vi "ConvertTriggerEventsToEventList.vi"(11 "Trigger Events":enum16{"Source", "Delay", "Sense", "None"}[](array[ring])) -> (3 "Event List":string)   [LabVIEW 2012, in "Keithley-6482.lvlib"]
uses:
  Keithley-6482.lvlib
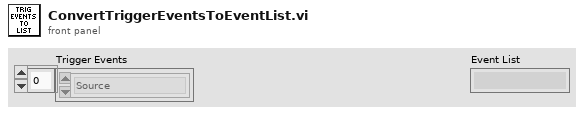
[diagram p1: front panel]
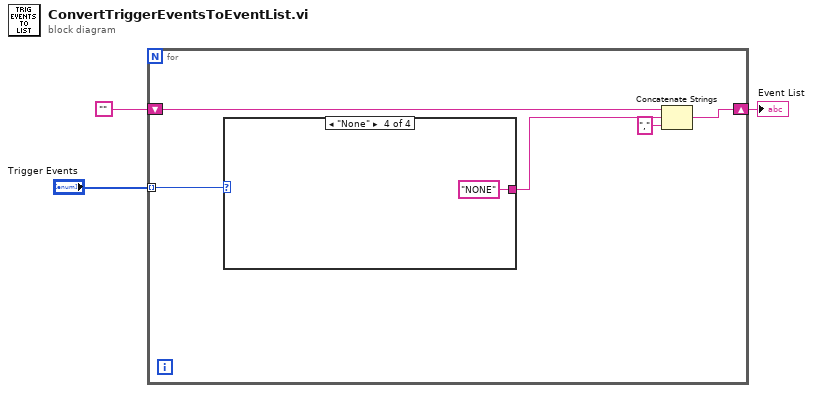
[diagram p0: block diagram]
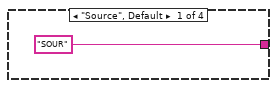
[diagram p2: hidden frame]
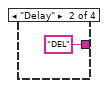
[diagram p3: hidden frame]
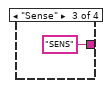
[diagram p4: hidden frame]
diagram:
  n1 = for {
    tunnel: "Trigger Events" -> [w6] mode=indexing
    shift-right: [w7] -> w1
    shift-left: "" -> [w8]
    n2 = case shown="\"None\"" w6 {
      tunnel: ["SOUR" "DEL" "SENS" "NONE"] -> w5
      frame "Source", Default {
      }
      frame "Delay" {
      }
      frame "Sense" {
      }
      frame "None" {
      }
    }
    n3 = Concatenate Strings(w8, w5, "," ("string")) -> (w7:string)
  }
  "Event List" <- w1
